vi "TestCloneAPI.vi"() -> ()   [LabVIEW 2018, in "ScopeModule.lvlib"]
uses:
  ScopeModule.lvlib
  TestInfo.ctl
  <userlib>/NIST/ModuleAdminLib/ModuleAdmin/ModuleAdmin.lvclass
  ScopeShared/Sync.ctl
  ScopeShared/clDidInit.ctl
  <userlib>/NIST/ModuleAdminLib/ModuleAdmin/ModuleAdmin.lvclass/ModuleAdmin.ctl
  ScopeShared/clStopArgument.ctl
  ScopeShared/Waveform.ctl
  ScopeShared/ScopeData.ctl
  <userlib>/NIST/ModuleAdminLib/ModuleAdmin/Accessors/Read CloneRegRef.vi
  <userlib>/NIST/ModuleAdminLib/CloneRegistration/CloneRegistration.lvclass
  ScopeShared/ScopeShared.lvlib
  Visualization/Visualization.lvlib
panel:
  in  "btnStopReading":bool
  in  "btnReadWaveform":bool
  in  "Tab Control":T1(tab)
  out "Waveform Graph":T2(graph)
  out "Waveform Chart":waveform(dbl)[](graph)
  out "Status Log":string
  in  "btnClear":bool
  in  "btnVisualization":bool caption="Visualization"
  out "Numeric Indicator":i32
  in  "SrcTerm":string(combo)="PFI1"
  in  "DestTerm":string(combo)="PXI_Trig2"
  in  "SyncHandle":refnum<k15>="PXI1Slot6"
  in  "btnSetSync":bool
  in  "btnClose":bool
  in  "btnConfigTrigger":bool
  in  "btnConfigChannels":bool
  in  "btnConfigAcquisition":bool
  in  "btnSettings":bool
  in  "btnInitialize":bool
  in  "btnAbort":bool
  in  "Show Panel":bool=TRUE
  in  "Plugin Type":u16(ring) items=["ScopeTest1"]
  in  "btnLoadPlugin":bool
  out "File Path Control":path
  in  "btnRequestINIPath":bool
  in  "btnRemove":bool
  out "Active Modules (Array)":string[](array[string])
  in  "btnAdd":bool
  in  "btnStop":bool
  in  "Select Module":i32(ring)=-1 caption="Select Module to send Request" items=["All"=-1]
  # "Hidden"
  # "Visible"
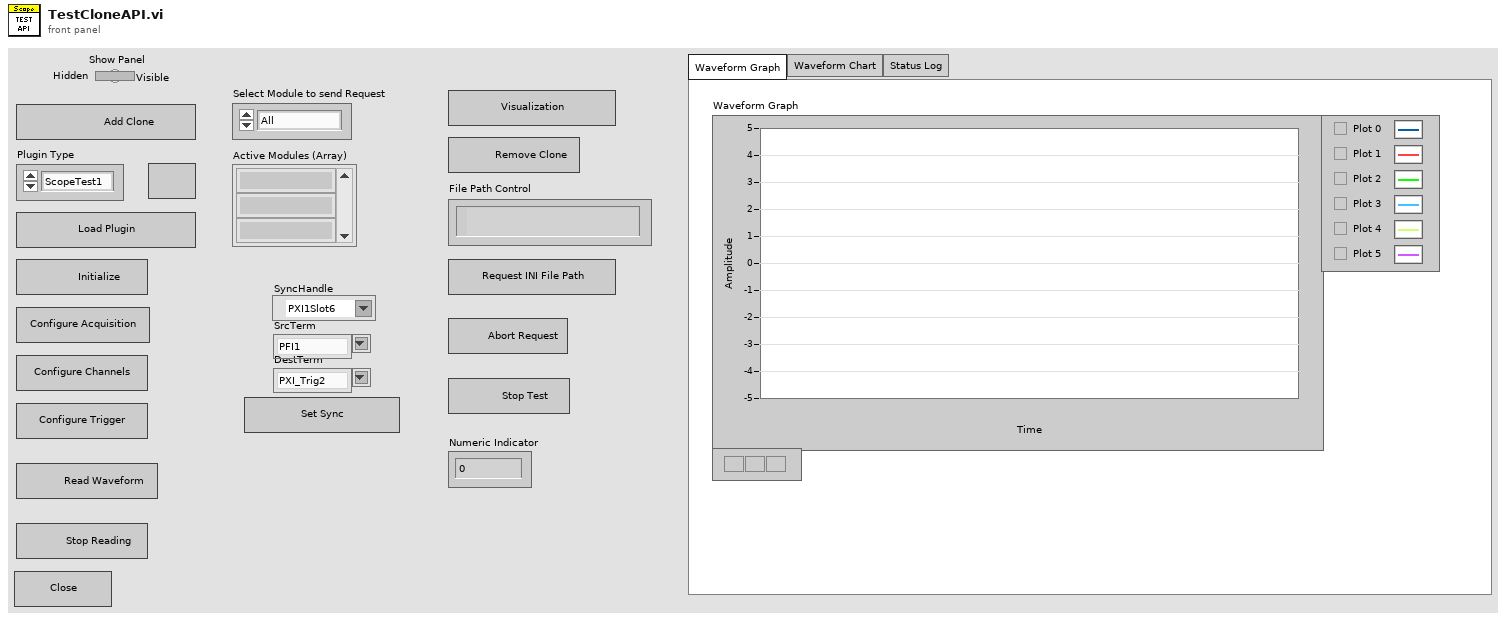
[diagram p1: front panel]
types:
  T1 = enum32{"Waveform Graph", "Waveform Chart", "Status Log"}
  T2 = cluster{"initial x":dbl, "x increment":dbl, "waveform array":dbl[]}[]
  T3 = typedef "ScopeModule.lvlib/TestInfo.ctl" = cluster{"PluginIniFilePaths":path[]}
  T4 = typedef "ScopeShared.lvlib/clBroadcastEvents.ctl" = cluster{"DidInit":refnum<user-event>, "StatusUpdate":refnum<user-event>, "ErrorReport":refnum<user-event>, "DidStop":refnum<user-event>, "PathToINI":refnum<user-event>, "Handle":refnum<user-event>, "Model":refnum<user-event>, "Channels":refnum<user-event>, "Acquisition":refnum<user-event>, "Trigger":refnum<user-event>, "ExtAcquisition":refnum<user-event>, "Waveform":refnum<user-event>}
  T5 = typedef "ScopeShared.lvlib/Sync.ctl" = cluster{"Handle":string, "SrcTerm":string, "DestTerm":string}
  T6 = typedef "ScopeShared.lvlib/clDidInit.ctl" = cluster{"Init?":bool, "ModuleAdmin":refnum<class "ModuleAdmin.lvclass">}
  T7 = typedef "ScopeShared.lvlib/clStopArgument.ctl" = cluster{"Exit via Stop Module Req?":bool, "Wait for Module to stop?":bool, "ModuleAdmin":refnum<class "ModuleAdmin.lvclass">}
  T8 = typedef "ScopeShared.lvlib/ScopeData.ctl" = cluster{"ScopeType":string, "ScopeData":variant}
  T9 = typedef "ScopeShared.lvlib/Waveform.ctl" = cluster{"initial x":dbl, "x increment":dbl, "waveform array":dbl[]}
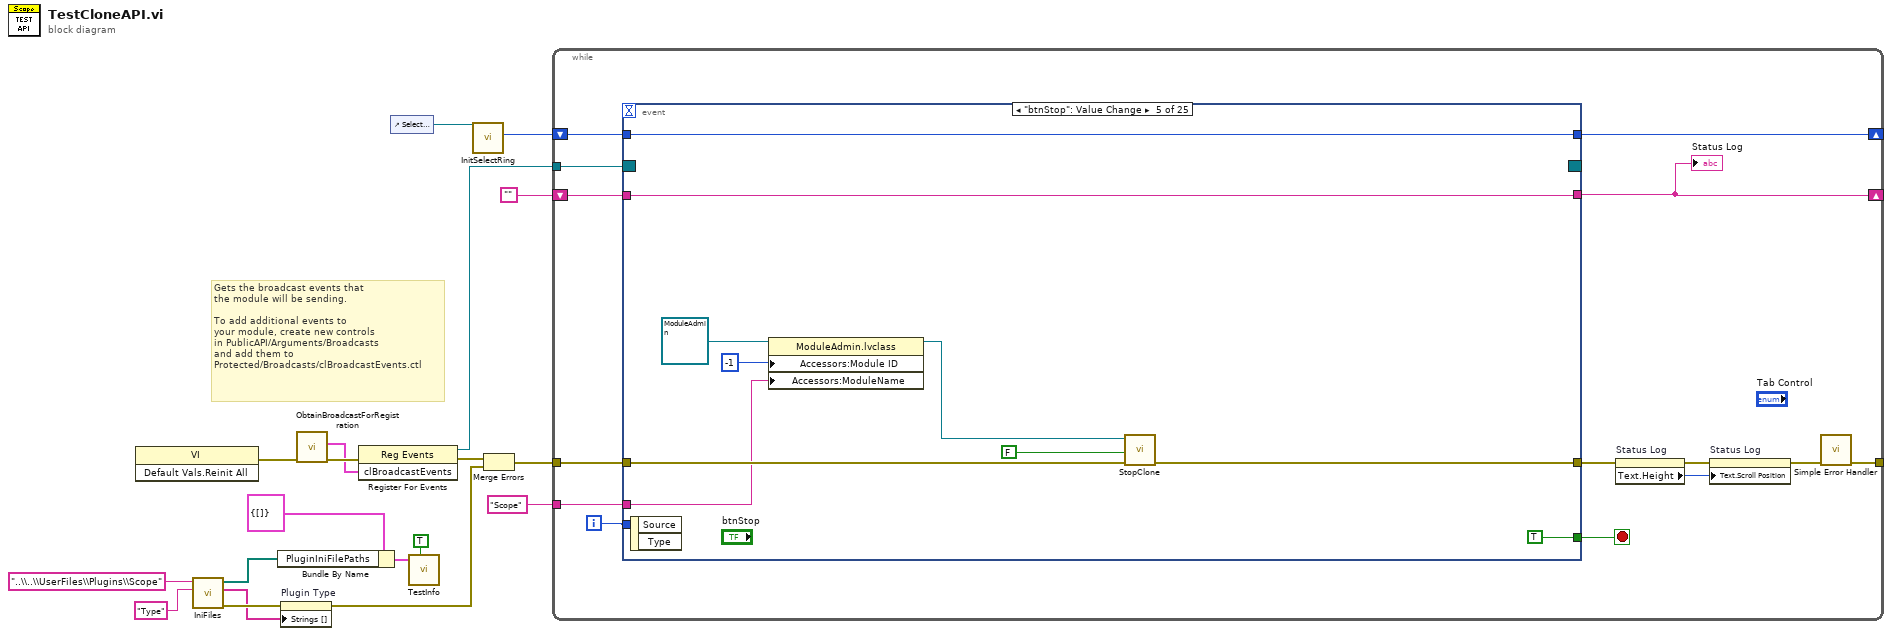
[diagram p0: block diagram]
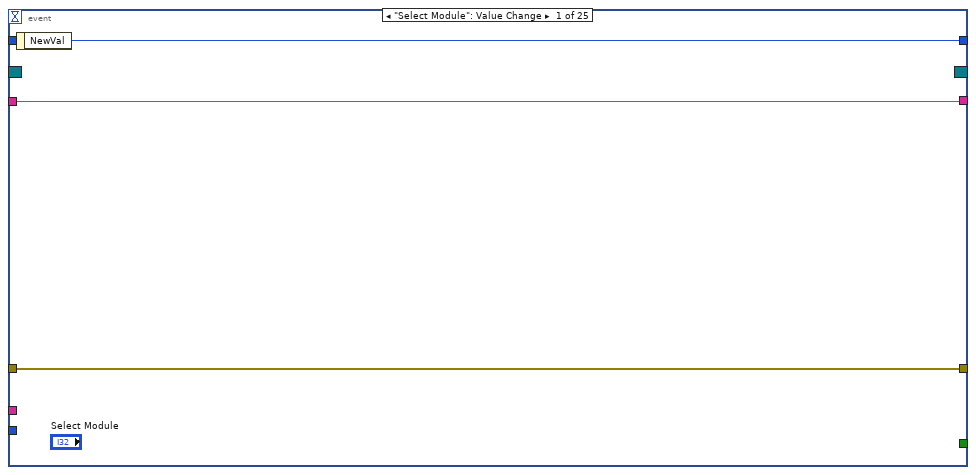
[diagram p2: hidden frame]
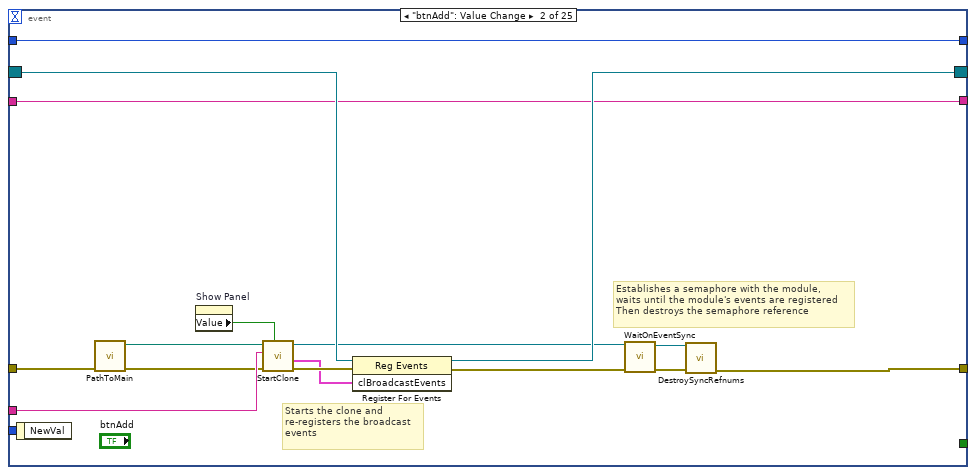
[diagram p3: hidden frame]
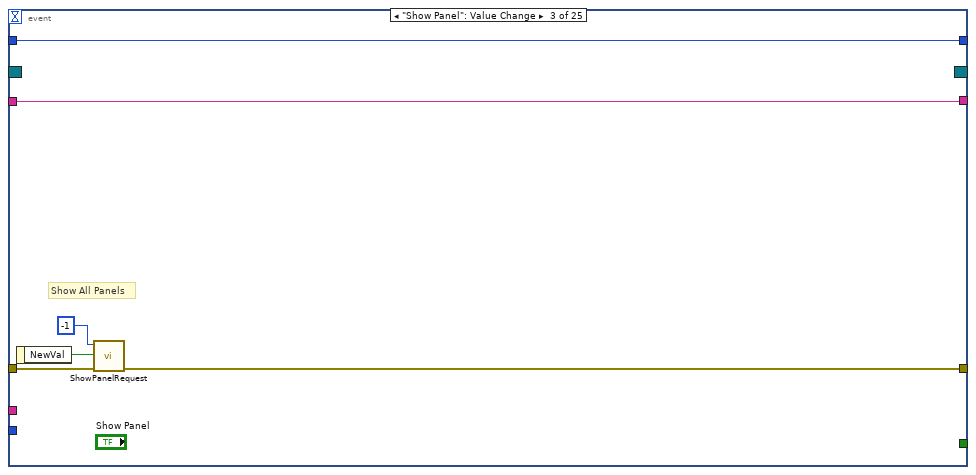
[diagram p4: hidden frame]
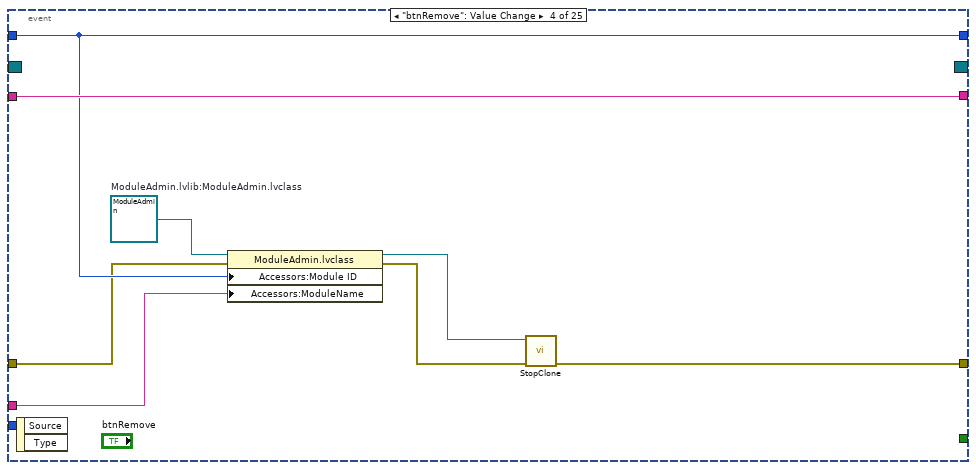
[diagram p5: hidden frame]
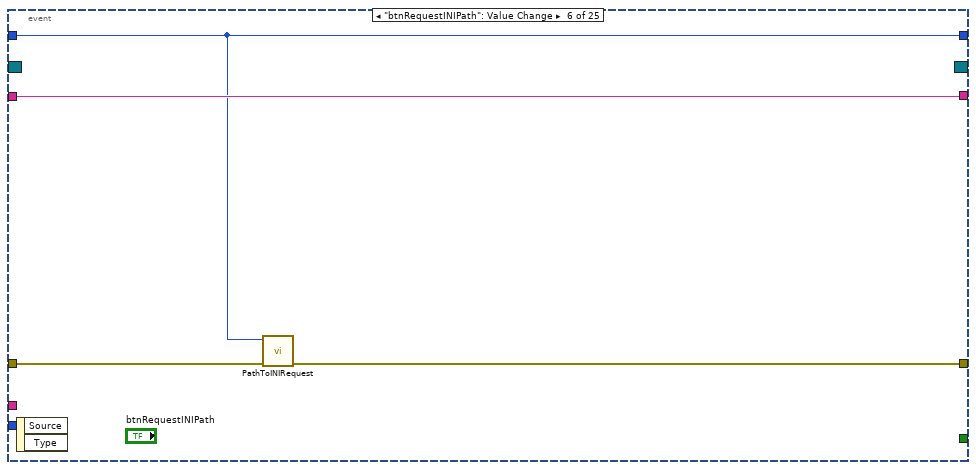
[diagram p6: hidden frame]
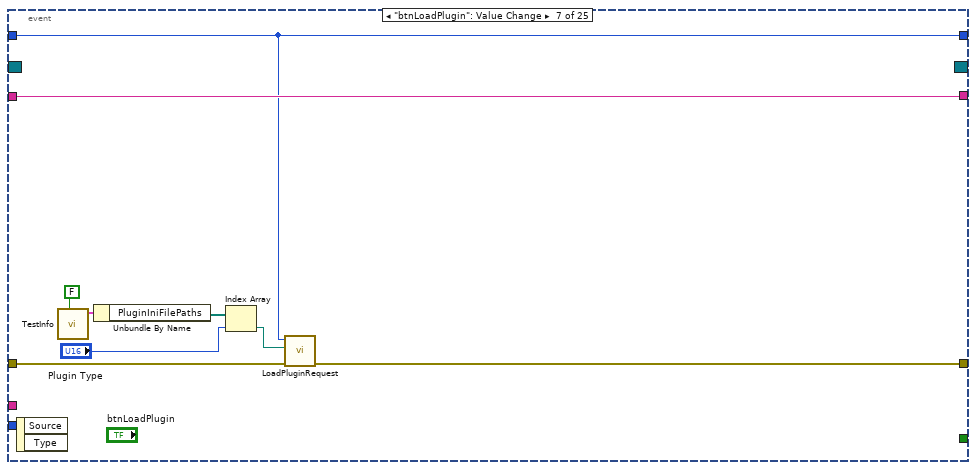
[diagram p7: hidden frame]
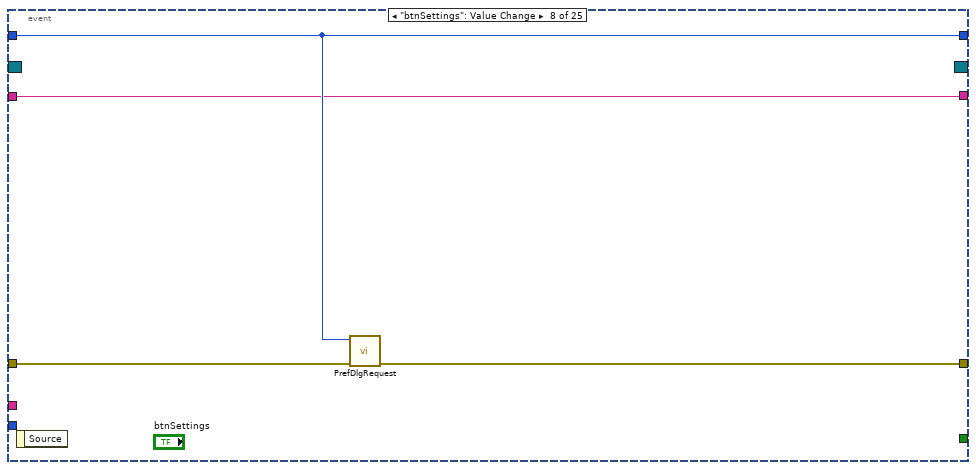
[diagram p8: hidden frame]
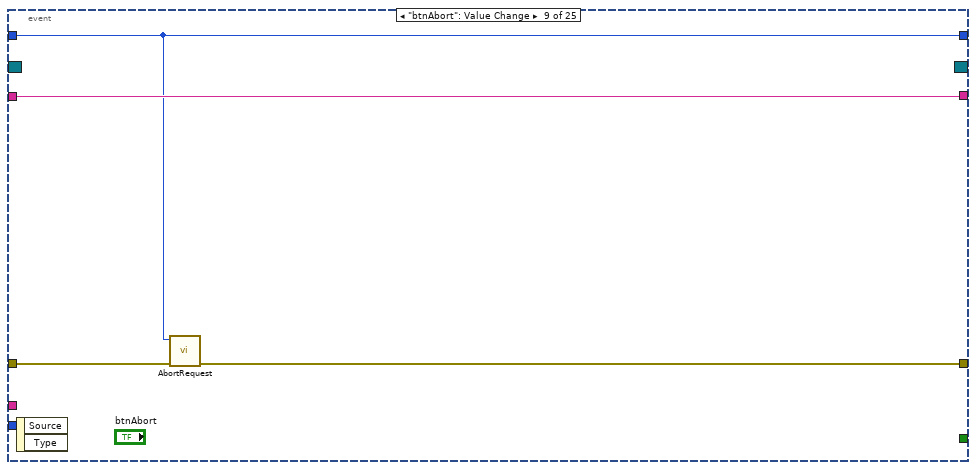
[diagram p9: hidden frame]
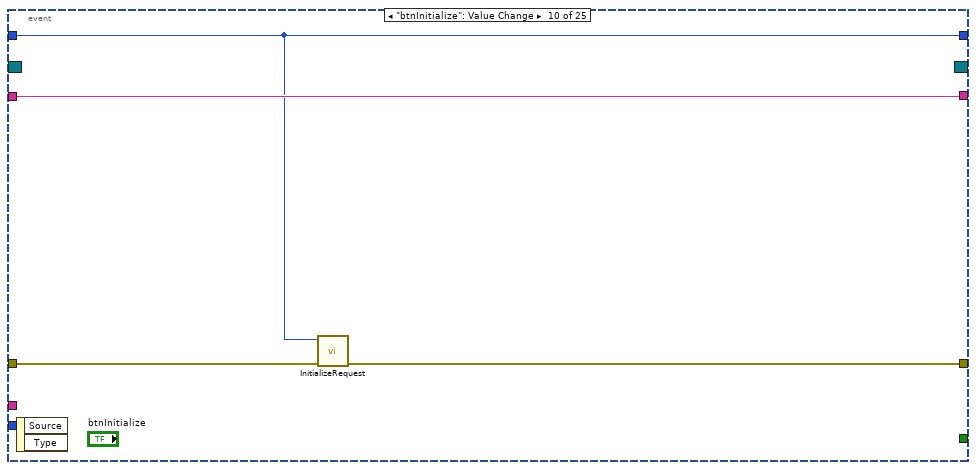
[diagram p10: hidden frame]
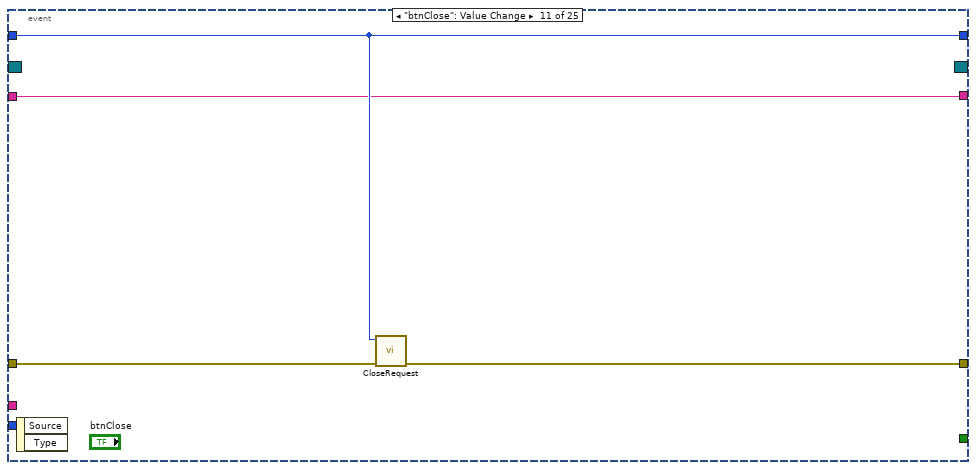
[diagram p11: hidden frame]
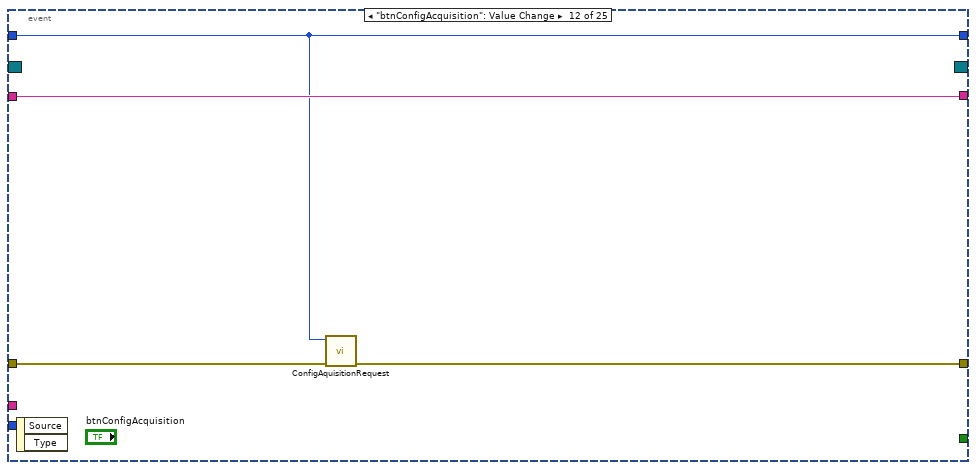
[diagram p12: hidden frame]
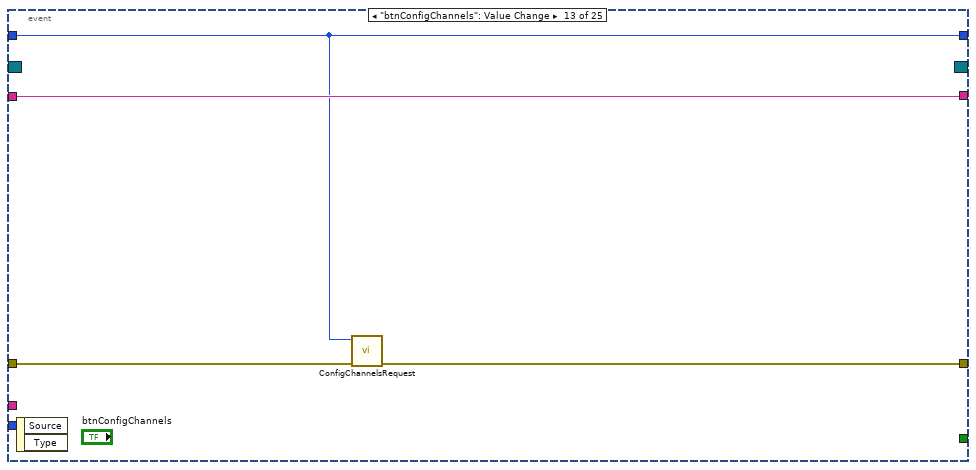
[diagram p13: hidden frame]
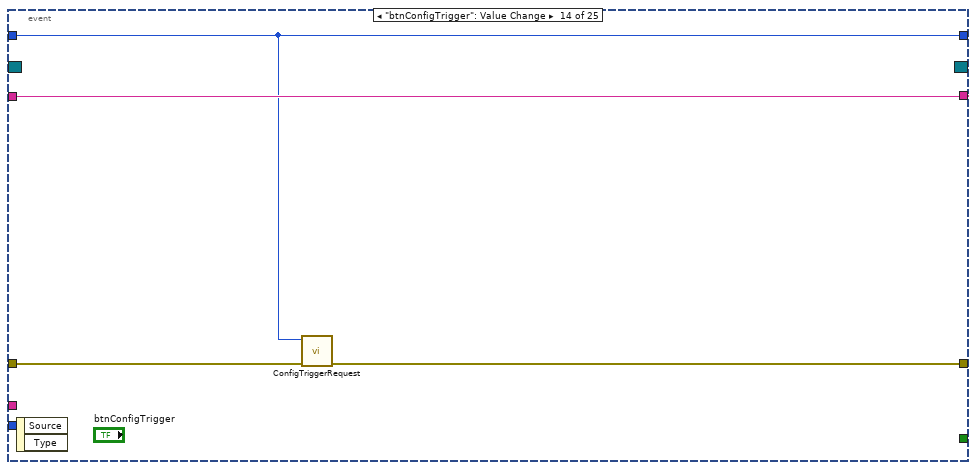
[diagram p14: hidden frame]
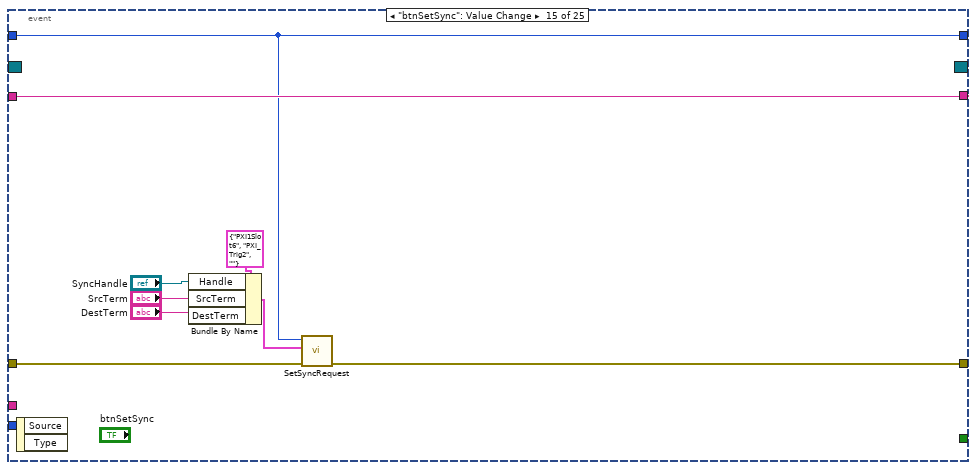
[diagram p15: hidden frame]
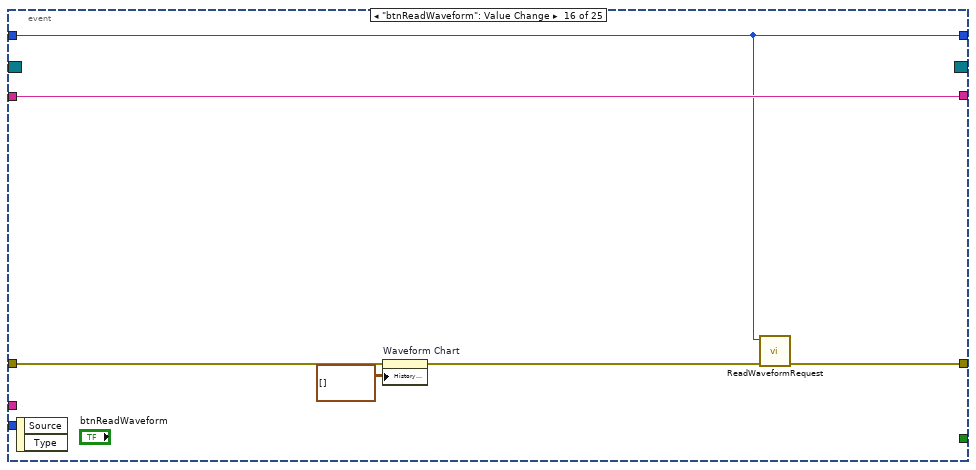
[diagram p16: hidden frame]
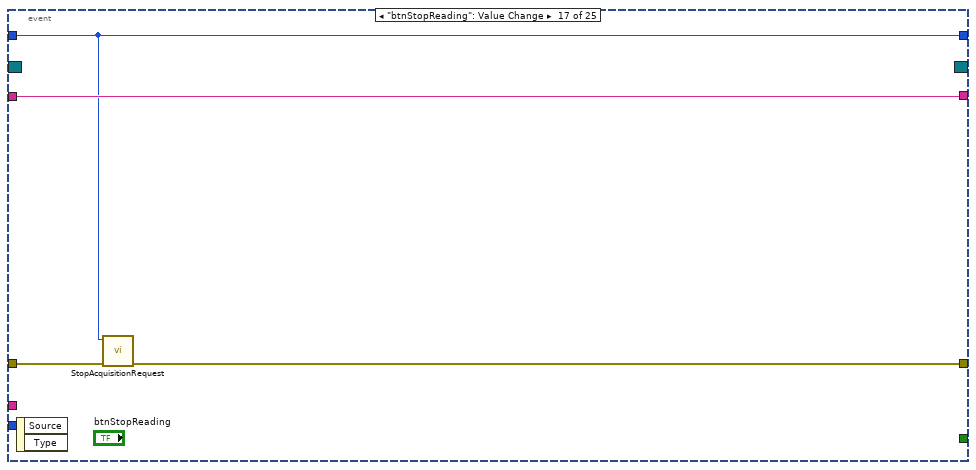
[diagram p17: hidden frame]
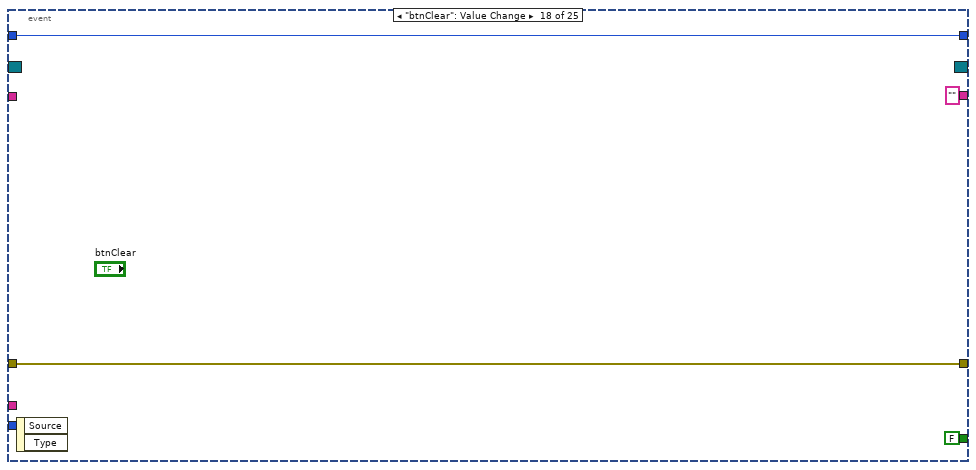
[diagram p18: hidden frame]
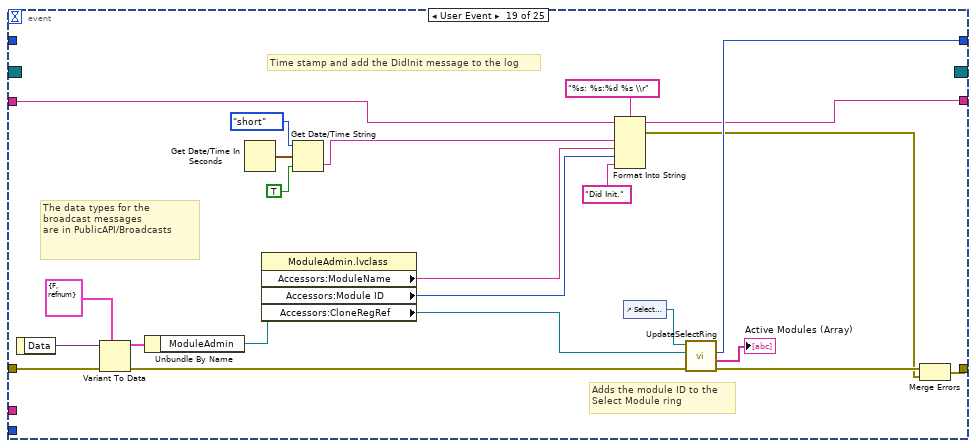
[diagram p19: hidden frame]
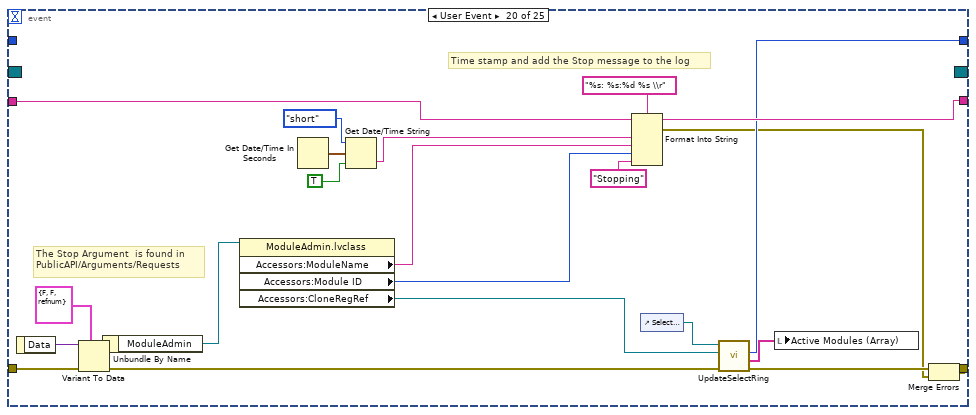
[diagram p20: hidden frame]
diagram:
  # "Gets the broadcast events that\nthe module will be sending.\n\nTo add additional events to\nyour module, create new controls\nin PublicAPI/Arguments/Broadcasts\nand add them to\nProtected/Broadcasts/clBroadcastEvents.ctl"
  n1 = invoke class="VI" method="Default Vals.Reinit All"() -> (error out=w17:errorcluster)  [unwired: 3 in, 2 out]
  n2 = call "IniFiles.vi"("iniKey"="Type", "name or relative path"="..\\..\\UserFiles\\Plugins\\Scope") -> ("error out"=w10:errorcluster, "Types"=w9:string[], "IniFilePaths"=w8:path[])  [unwired: 7 in]
  n3 = Bundle By Name(cluster=T3 {"PluginIniFilePaths"=[]} ("TestInfo"), "PluginIniFilePaths"=w8) -> (w7:T3)
  n4 = property on="Plugin Type" class="Ring (strict)"(error in=w10, "Strings []"=w9) -> (error out=w1:errorcluster)  [unwired: 1 in, 1 out]
  n5 = call "ObtainBroadcastForRegistration.vi"("error in (no error)"=w17) -> ("error out"=w16:errorcluster, "clBroadcastEvents"=w15:T4)  [unwired: 9 in]
  n6 = register-events(error in=w16, w15) -> (reference out=w13:refnum<event-registration>, error out=w14:errorcluster)  [unwired: 1 in]
  n7 = control-ref of="Select Module"() -> (w19:refnum<vi>)
  n8 = call "TestInfo.vi"("Set (f)"=TRUE, "TestInfo 2"=w7) -> ()  [unwired: 9 in, 1 out]
  n9 = call "InitSelectRing.vi"("Ring Refnum"=w19) -> ("Module Ring Value"=w18:i32)  [unwired: 9 in, 1 out]
  n10 = Merge Errors(w14, w1) -> (w5:errorcluster)
  n11 = while {
    shift-right: [w32] -> _
    shift-left: w18 -> [w33]
    tunnel: w5 -> [w30]
    tunnel: w13 -> [w28]
    tunnel: [w29] -> _
    shift-right: [w27] -> _
    shift-left: "" -> [w26]
    tunnel: "Scope" ("ModuleName") -> [w25]
    i -> [w22]
    stop <- w31 stop-if-true
    n12 = event shown="[4] \"btnStop\": Value Change" {
      selector: w28 -> [_ w45 _ _ _ _ _ _ _ _ _ _ _ _ _ _ _ _ _ _ _ _ _ _ _]
      dyn-events: [_ w44 _ _ _ _ _ _ _ _ _ _ _ _ _ _ _ _ _ _ _ _ _ _ _] -> _
      timeout: _ -> [_ _ _ _ _ _ _ _ _ _ _ _ _ _ _ _ _ _ _ _ _ _ _ _ _]
      tunnel: w33 -> [_ w52 w54 w63 w76 w79 w82 w91 w94 w99 w103 w106 w110 w114 w123 w131 w135 w137 _ _ w201 w205 w216 w226 w241]
      tunnel: [w36 w52 w54 w63 w76 w79 w82 w91 w94 w99 w103 w106 w110 w114 w123 w131 w135 w137 w158 w173 w201 w205 w216 w226 w241] -> w32
      tunnel: [_ _ _ _ TRUE _ _ _ _ _ _ _ _ _ _ _ _ FALSE _ _ _ _ _ _ _] -> w31
      tunnel: w30 -> [w34 w39 w57 w60 w74 w78 w88 w93 w97 w101 w105 w108 w113 w117 w126 w129 w134 w140 w163 w182 w198 w209 w212 w229 _]
      tunnel: [w34 w46 w55 w65 w72 w77 w81 w92 w95 w98 w104 w107 w112 w116 w125 w130 w133 w140 w147 w170 w192 w208 w211 w222 w238] -> w21
      tunnel: [w35 w43 w53 w66 w71 w80 w89 w90 w96 w100 w102 w109 w111 w115 w124 w132 w136 "" w151 w179 w195 w204 w217 w227 w242] -> w27
      tunnel: w26 -> [w35 w43 w53 w66 w71 w80 w89 w90 w96 w100 w102 w109 w111 w115 w124 w132 w136 _ w150 w180 w200 w204 w217 w227 w242]
      tunnel: w25 -> [_ w42 _ w62 w68 _ _ _ _ _ _ _ _ _ _ _ _ _ _ _ _ _ _ _ _]
      tunnel: w22 -> [_ _ _ _ _ _ _ _ _ _ _ _ _ _ _ _ _ _ _ _ _ _ _ w225 _]
      event "Select Module": Value Change {
        n13 = event-data() -> ("NewVal"=w36:i32)  [unwired: 1 in]
      }
      event "btnAdd": Value Change {
        # "Establishes a semaphore with the module,\nwaits until the module's events are registered\nThen destroys the semaphore reference"
        # "Starts the clone and\nre-registers the broadcast \nevents"
        n14 = event-data() -> ()  [unwired: 1 in, 1 out]
        n15 = call "PathToMain.vi"("Error In"=w39) -> ("Error Out"=w38:errorcluster, "PathToMain"=w37:path)  [unwired: 9 in]
        n16 = property on="Show Panel" class="Bool (strict)"() -> ("Value"=w40:bool)  [unwired: 2 in, 2 out]
        n17 = call "StartClone.vi"("ShowPanel? (f)"=w40, "error in (no error)"=w38, "ModuleName"=w42, "vi path"=w37) -> ("error out"=w51:errorcluster, "clBroadcastEvents"=w47:T4, "ModuleAdmin"=w41:refnum<class "ModuleAdmin.lvclass">)  [unwired: 5 in]
        n18 = register-events(reference=w45, error in=w51, w47) -> (reference out=w44:refnum<event-registration>, error out=w50:errorcluster)
        n19 = call <userlib>:"WaitOnEventSync.vi"("error in (no error)"=w50, "ModuleAdmin"=w41) -> ("error out"=w49:errorcluster, "ModuleAdmin"=w48:refnum<class "ModuleAdmin.lvclass">)  [unwired: 8 in]
        n20 = call <userlib>:"DestroySyncRefnums.vi"("error in (no error)"=w49, "ModuleAdmin"=w48) -> ("error out"=w46:errorcluster)  [unwired: 9 in]
      }
      event "Show Panel": Value Change {
        # "Show All Panels"
        n21 = event-data() -> ("NewVal"=w58:bool)  [unwired: 1 in]
        n22 = call "ShowPanelRequest.vi"("error in (no error)"=w57, "ShowPanel?"=w58, "ModuleID"=-1) -> ("error out"=w55:errorcluster)  [unwired: 8 in]
      }
      event "btnRemove": Value Change {
        w64 = refnum<class "ModuleAdmin.lvclass"> refnum  # ModuleAdmin.lvlib:ModuleAdmin.lvclass
        n23 = event-data() -> ()  [unwired: 1 in, 2 out]
        n24 = property class="ModuleAdmin.lvclass"(reference=w64, error in=w60, "Accessors:Module ID"=w63, "Accessors:ModuleName"=w62) -> (reference out=w61:refnum<class "ModuleAdmin.lvclass">, error out=w59:errorcluster)
        n25 = call "StopClone.vi"("error in (no error)"=w59, "ModuleAdmin"=w61) -> ("error out"=w65:errorcluster)  [unwired: 9 in]
      }
      event "btnStop": Value Change {
        n26 = event-data() -> ()  [unwired: 1 in, 2 out]
        n27 = property class="ModuleAdmin.lvclass"(reference=refnum<class "ModuleAdmin.lvclass"> refnum ("ModuleAdmin.lvlib:ModuleAdmin.lvclass"), "Accessors:Module ID"=-1 ("Module ID"), "Accessors:ModuleName"=w68) -> (reference out=w67:refnum<class "ModuleAdmin.lvclass">)  [unwired: 1 in, 1 out]
        n28 = call "StopClone.vi"("error in (no error)"=w74, "Wait for Module to stop?"=FALSE, "ModuleAdmin"=w67) -> ("error out"=w72:errorcluster)  [unwired: 8 in]
      }
      event "btnRequestINIPath": Value Change {
        n29 = event-data() -> ()  [unwired: 1 in, 2 out]
        n30 = call "PathToINIRequest.vi"("error in (no error)"=w78, "ModuleID"=w79) -> ("error out"=w77:errorcluster)  [unwired: 9 in]
      }
      event "btnLoadPlugin": Value Change {
        n31 = event-data() -> ()  [unwired: 1 in, 2 out]
        n32 = call "TestInfo.vi"("Set (f)"=FALSE) -> ("TestInfo"=w86:T3)  [unwired: 10 in]
        n33 = Unbundle By Name(w86) -> ("PluginIniFilePaths"=w85:path[])
        n34 = Index Array(array=w85, index="Plugin Type") -> (element=w83:path)
        n35 = call "LoadPluginRequest.vi"("error in (no error)"=w88, "PathToPluginINI"=w83, "ModuleID"=w82) -> ("error out"=w81:errorcluster)  [unwired: 8 in]
      }
      event "btnSettings": Value Change {
        n36 = event-data() -> ()  [unwired: 1 in, 1 out]
        n37 = call "PrefDlgRequest.vi"("error in (no error)"=w93, "ModuleID"=w91) -> ("error out"=w92:errorcluster)  [unwired: 9 in]
      }
      event "btnAbort": Value Change {
        n38 = event-data() -> ()  [unwired: 1 in, 2 out]
        n39 = call "AbortRequest.vi"("error in (no error)"=w97, "ModuleID"=w94) -> ("error out"=w95:errorcluster)  [unwired: 9 in]
      }
      event "btnInitialize": Value Change {
        n40 = event-data() -> ()  [unwired: 1 in, 2 out]
        n41 = call "InitializeRequest.vi"("error in (no error)"=w101, "ModuleID"=w99) -> ("error out"=w98:errorcluster)  [unwired: 9 in]
      }
      event "btnClose": Value Change {
        n42 = event-data() -> ()  [unwired: 1 in, 2 out]
        n43 = call "CloseRequest.vi"("error in (no error)"=w105, "ModuleID"=w103) -> ("error out"=w104:errorcluster)  [unwired: 9 in]
      }
      event "btnConfigAcquisition": Value Change {
        n44 = event-data() -> ()  [unwired: 1 in, 2 out]
        n45 = call "ConfigAquisitionRequest.vi"("error in (no error)"=w108, "ModuleID"=w106) -> ("error out"=w107:errorcluster)  [unwired: 9 in]
      }
      event "btnConfigChannels": Value Change {
        n46 = event-data() -> ()  [unwired: 1 in, 2 out]
        n47 = call "ConfigChannelsRequest.vi"("error in (no error)"=w113, "ModuleID"=w110) -> ("error out"=w112:errorcluster)  [unwired: 9 in]
      }
      event "btnConfigTrigger": Value Change {
        n48 = event-data() -> ()  [unwired: 1 in, 2 out]
        n49 = call "ConfigTriggerRequest.vi"("error in (no error)"=w117, "ModuleID"=w114) -> ("error out"=w116:errorcluster)  [unwired: 9 in]
      }
      event "btnSetSync": Value Change {
        n50 = event-data() -> ()  [unwired: 1 in, 2 out]
        n51 = Bundle By Name(cluster=T5 {"Handle"="PXI1Slot6", "SrcTerm"="PXI_Trig2", "DestTerm"=""} ("Sync"), "Handle"="SyncHandle", "SrcTerm"="SrcTerm", "DestTerm"="DestTerm") -> (w120:T5)
        n52 = call "SetSyncRequest.vi"("error in (no error)"=w126, "Sync"=w120, "ModuleID"=w123) -> ("error out"=w125:errorcluster)  [unwired: 8 in]
      }
      event "btnReadWaveform": Value Change {
        n53 = event-data() -> ()  [unwired: 1 in, 2 out]
        n54 = property on="Waveform Chart" class="WFChart (strict)"(error in=w129, "History Data"=waveform(dbl)[][] []) -> (error out=w128:errorcluster)  [unwired: 1 in, 1 out]
        n55 = call "ReadWaveformRequest.vi"("error in (no error)"=w128, "ModuleID"=w131) -> ("error out"=w130:errorcluster)  [unwired: 9 in]
      }
      event "btnStopReading": Value Change {
        n56 = event-data() -> ()  [unwired: 1 in, 2 out]
        n57 = call "StopAcquisitionRequest.vi"("error in (no error)"=w134, "ModuleID"=w135) -> ("error out"=w133:errorcluster)  [unwired: 9 in]
      }
      event "btnClear": Value Change {
        n58 = event-data() -> ()  [unwired: 1 in, 2 out]
      }
      event User Event {
        # "Adds the module ID to the \nSelect Module ring"
        # "Time stamp and add the DidInit message to the log"
        # "The data types for the broadcast messages\nare in PublicAPI/Broadcasts"
        n59 = event-data() -> ("Data"=w162:variant)  [unwired: 1 in]
        n60 = Variant To Data(error in=w163, type=T6 {"Init?"=FALSE, "ModuleAdmin"=refnum} ("clDidInit"), Variant=w162) -> (data=w155:T6, error out=w160:errorcluster)
        n61 = Unbundle By Name(w155) -> ("ModuleAdmin"=w145:refnum<class "ModuleAdmin.lvclass">)
        n62 = Get Date/Time In Seconds() -> (seconds since 1Jan1904=w153:timestamp)
        n63 = property class="ModuleAdmin.lvclass"(reference=w145) -> ("Accessors:ModuleName"=w143:string, "Accessors:Module ID"=w142:i32, "Accessors:CloneRegRef"=w141:refnum<data-value>)  [unwired: 1 in, 2 out]
        n64 = Get Date/Time String(date format (0)=enum16{"short", "long", "abbreviated"}."short", seconds (now)=w153, want seconds? (F)=TRUE) -> (time string=w156:string)  [unwired: 1 out]
        n65 = Format Into String(format string="%s: %s:%d %s \\r", initial string=w150, w156, w143, w142, "Did Init.") -> (resulting string=w151:string, error out=w148:errorcluster)  [unwired: 1 in]
        n66 = control-ref of="Select Module"() -> (w159:refnum<vi>)
        n67 = call "UpdateSelectRing.vi"("error in (no error)"=w160, "CloneRegRef"=w141, "Ring Refnum"=w159) -> ("error out"=w149:errorcluster, "ActiveModules"=→"Active Modules (Array)":string[], "Module Ring Value"=w158:i32)  [unwired: 6 in]
        n68 = Merge Errors(w149, w148) -> (w147:errorcluster)
      }
      event User Event {
        # "Time stamp and add the Stop message to the log"
        # "The Stop Argument  is found in\nPublicAPI/Arguments/Requests"
        n69 = event-data() -> ("Data"=w181:variant)  [unwired: 1 in]
        n70 = Variant To Data(error in=w182, type=T7 {"Exit via Stop Module Req?"=FALSE, "Wait for Module to stop?"=FALSE, "ModuleAdmin"=refnum} ("Stop Argument"), Variant=w181) -> (data=w177:T7, error out=w176:errorcluster)
        n71 = Unbundle By Name(w177) -> ("ModuleAdmin"=w168:refnum<class "ModuleAdmin.lvclass">)
        n72 = property class="ModuleAdmin.lvclass"(reference=w168) -> ("Accessors:ModuleName"=w166:string, "Accessors:Module ID"=w165:i32, "Accessors:CloneRegRef"=w164:refnum<data-value>)  [unwired: 1 in, 2 out]
        n73 = Get Date/Time In Seconds() -> (seconds since 1Jan1904=w184:timestamp)
        n74 = Get Date/Time String(date format (0)=enum16{"short", "long", "abbreviated"}."short", seconds (now)=w184, want seconds? (F)=TRUE) -> (time string=w186:string)  [unwired: 1 out]
        n75 = Format Into String(format string="%s: %s:%d %s \\r", initial string=w180, w186, w166, w165, "Stopping") -> (resulting string=w179:string, error out=w171:errorcluster)  [unwired: 1 in]
        n76 = control-ref of="Select Module"() -> (w175:refnum<vi>)
        n77 = call "UpdateSelectRing.vi"("error in (no error)"=w176, "CloneRegRef"=w164, "Ring Refnum"=w175) -> ("error out"=w172:errorcluster, "ActiveModules"=w174:string[], "Module Ring Value"=w173:i32)  [unwired: 6 in]
        n78 = local write "Active Modules (Array)"(w174) -> ()
        n79 = Merge Errors(w172, w171) -> (w170:errorcluster)
      }
      event User Event {
        # "Time stamp and add the Status message to the log"
        # "The data types for the broadcast messages\nare in PublicAPI/Broadcasts"
        n80 = event-data() -> ("Data"=w197:variant)  [unwired: 1 in]
        n81 = Variant To Data(error in=w198, type="", Variant=w197) -> (data=w187:string, error out=w194:errorcluster)
        n82 = Get Date/Time In Seconds() -> (seconds since 1Jan1904=w196:timestamp)
        n83 = Get Date/Time String(date format (0)=enum16{"short", "long", "abbreviated"}."short", seconds (now)=w196, want seconds? (F)=TRUE) -> (time string=w189:string)  [unwired: 1 out]
        n84 = Format Into String(format string="%s: %s \\r", initial string=w200, w189, w187) -> (resulting string=w195:string, error out=w193:errorcluster)  [unwired: 1 in]
        n85 = Merge Errors(w194, w193) -> (w192:errorcluster)
      }
      event User Event {
        # "#CodeNeeded\nThis is a very crude error handler\nA better error handler will be needed"
        # "The data types for the broadcast messages\nare in PublicAPI/Broadcasts"
        n86 = event-data() -> ("ModuleID"=w207:i32, "Data"=w210:variant)  [unwired: 1 in]
        n87 = Variant To Data(error in=w209, type=errorcluster {"status"=FALSE, "code"=0, "source"=""} ("error constant"), Variant=w210) -> (data=w202:errorcluster, error out=w208:errorcluster)
        n88 = Number To Decimal String(number=w207) -> (decimal integer string=w206:string)  [unwired: 1 in]
        n89 = call <vilib>:"General Error Handler.vi"("[error source] (\" \")"=w206, "error in (no error)"=w202) -> ()  [unwired: 9 in, 5 out]
      }
      event User Event {
        n90 = event-data() -> ("Data"=w214:variant)  [unwired: 1 in, 1 out]
        n91 = Variant To Data(error in=w212, type=path "" ("Path"), Variant=w214) -> (data=→"File Path Control":path, error out=w211:errorcluster)
      }
      event User Event {
        n92 = event-data() -> ("Data"=w228:variant)  [unwired: 1 in]
        n93 = Variant To Data(error in=w229, type=T8 {"ScopeType"="", "ScopeData"=variant} ("ScopeData"), Variant=w228) -> (data=w219:T8, error out=w223:errorcluster)
        n94 = Unbundle By Name(w219) -> ("ScopeData"=w218:variant)
        n95 = Variant To Data(error in=w223, type=T9[] [], Variant=w218) -> (data=w220:T9[], error out=w222:errorcluster)
        "Waveform Graph" <- w220
        n96 = disable-structure shown="Enabled" {
          disable-tunnel: w220 -> [w231 _]
          frame Enabled {
            n97 = for {
              tunnel: w231 -> [w237] mode=indexing
              tunnel: [w232] -> w230 mode=indexing
              n98 = Unbundle By Name(w237) -> ("initial x"=w235:dbl, "x increment"=w234:dbl, "waveform array"=w233:dbl[])
              n99 = To Time Stamp(1:w235) -> (0:w236:timestamp)
              n100 = Bundle By Name("t0"=w236, "dt"=w234, "Y"=w233) -> (w232:waveform(dbl))  [unwired: 1 in]
            }
            "Waveform Chart" <- w230
          }
          frame Disabled {
          }
        }
        "Numeric Indicator" <- w225
      }
      event "btnVisualization": Value Change {
        n101 = event-data() -> ()  [unwired: 1 in, 2 out]
        n102 = call "dlgSelectVisApps.vi"("PathsToVisApps"=string[] ["VisualizeStatus", "VisualizeScope"]) -> ("Error Out"=w239:errorcluster[])  [unwired: 10 in]
        n103 = Merge Errors(w239) -> (w238:errorcluster)
      }
    }
    "Status Log" <- w27
    n104 = property on="Status Log" class="Str"(error in=w21) -> (error out=w20:errorcluster, "Text.Height"=w23:u32)  [unwired: 1 in, 1 out]
    n105 = property on="Status Log" class="Str"(error in=w20, "Text.Scroll Position"=w23) -> (error out=w24:errorcluster)  [unwired: 1 in, 1 out]
    n106 = call <vilib>:"Simple Error Handler.vi"("error in (no error)"=w24) -> ("error out"=w29:errorcluster)  [unwired: 4 in, 4 out]
  }
